vi "Test Plan - Remove Empty Element (SubVI).vi"(11 "Data":string[](array[string])) -> (3 "Result":string[](array[string]))   [LabVIEW 2019]
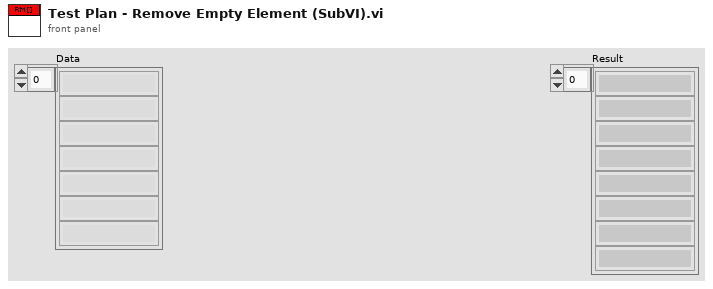
[diagram p1: front panel]
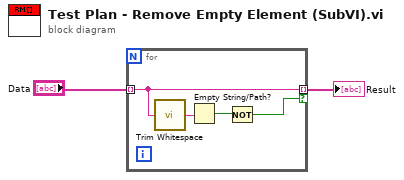
[diagram p0: block diagram]
diagram:
  n1 = for {
    tunnel: "Data" -> [w4] mode=indexing
    tunnel: [w4] -> w2 mode=indexing if=w3
    n2 = call <vilib>:"Trim Whitespace.vi"("string"=w4) -> ("trimmed string"=w6:string)  [unwired: 1 in]
    n3 = Empty String/Path?(string/path=w6) -> (empty?=w5:bool)
    n4 = Not(x=w5) -> (.not. x?=w3:bool)
  }
  "Result" <- w2
